vi "Main IU.vi"() -> ()   [LabVIEW 2019]
panel:
  out "Numeric":dbl
  in  "RESET 2":bool
  in  "Tiempo 2":dbl
  in  "Tiempo 1":dbl
  in  "Home":bool
  in  "Aceleración final Motor 2":dbl
  in  "Aceleración final Motor 1":dbl
  in  "Velocidad final Motor 2":dbl
  in  "Velocidad final Motor 1":dbl
  out "String":string
  in  "GO 2":bool
  in  "Aceleración inicial Motor 2":dbl
  in  "Aceleración inicial Motor 1":dbl
  in  "Velocidad inicial Motor 2":dbl
  in  "Velocidad inicial Motor 1":dbl
  in  "RESET 1":bool
  in  "Trayectoria":bool
  in  "GO":bool
  in  "Posición final Motor 2":dbl
  in  "MOTORES INDEPENDIENTES":bool
  in  "Tab Control":enum32{"Motor 1", "Motor 2"}(tab)
  out "Waveform Chart 6":waveform(dbl)[](graph)
  out "Waveform Chart 5":waveform(dbl)[](graph)
  out "Hall 1":bool
  out "Hall 2":bool
  out "Waveform Chart 4":waveform(dbl)[](graph)
  out "Waveform Chart 3":waveform(dbl)[](graph)
  out "Hall 2":bool
  out "Waveform Chart 2":waveform(dbl)[](graph)
  out "Hall1":bool
  in  "Stop UI and RT":bool
  in  "Stop UI":bool
  in  "Posición final motor 1":dbl
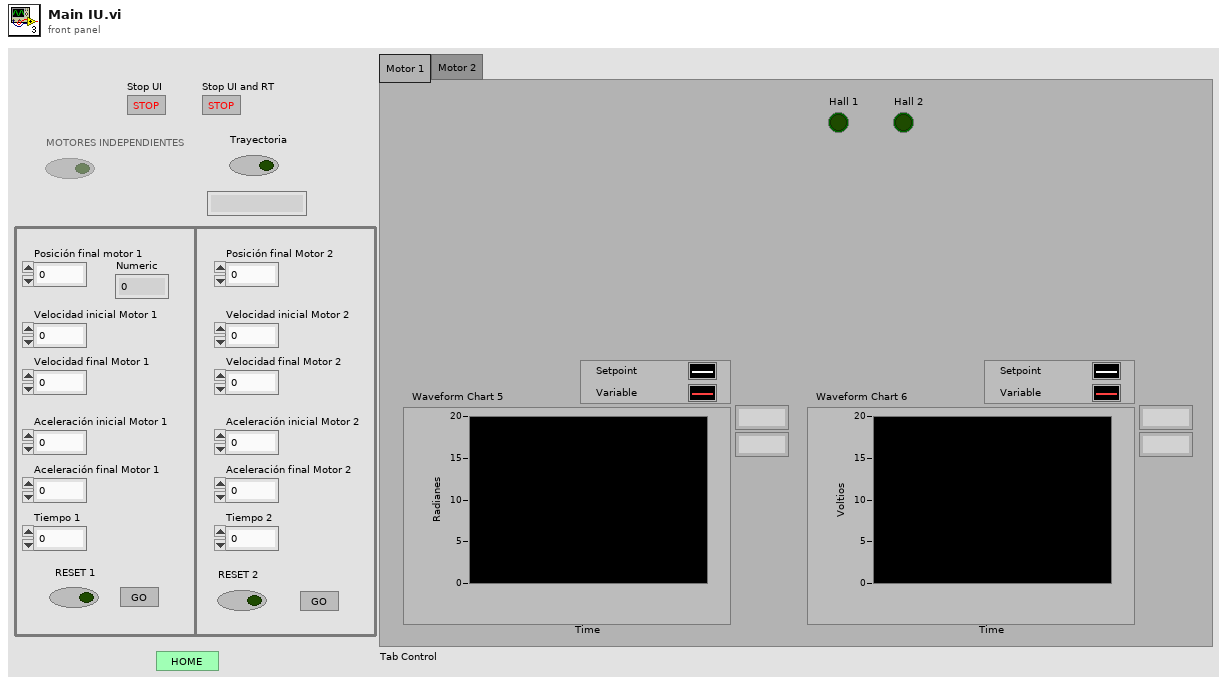
[diagram p1: front panel]
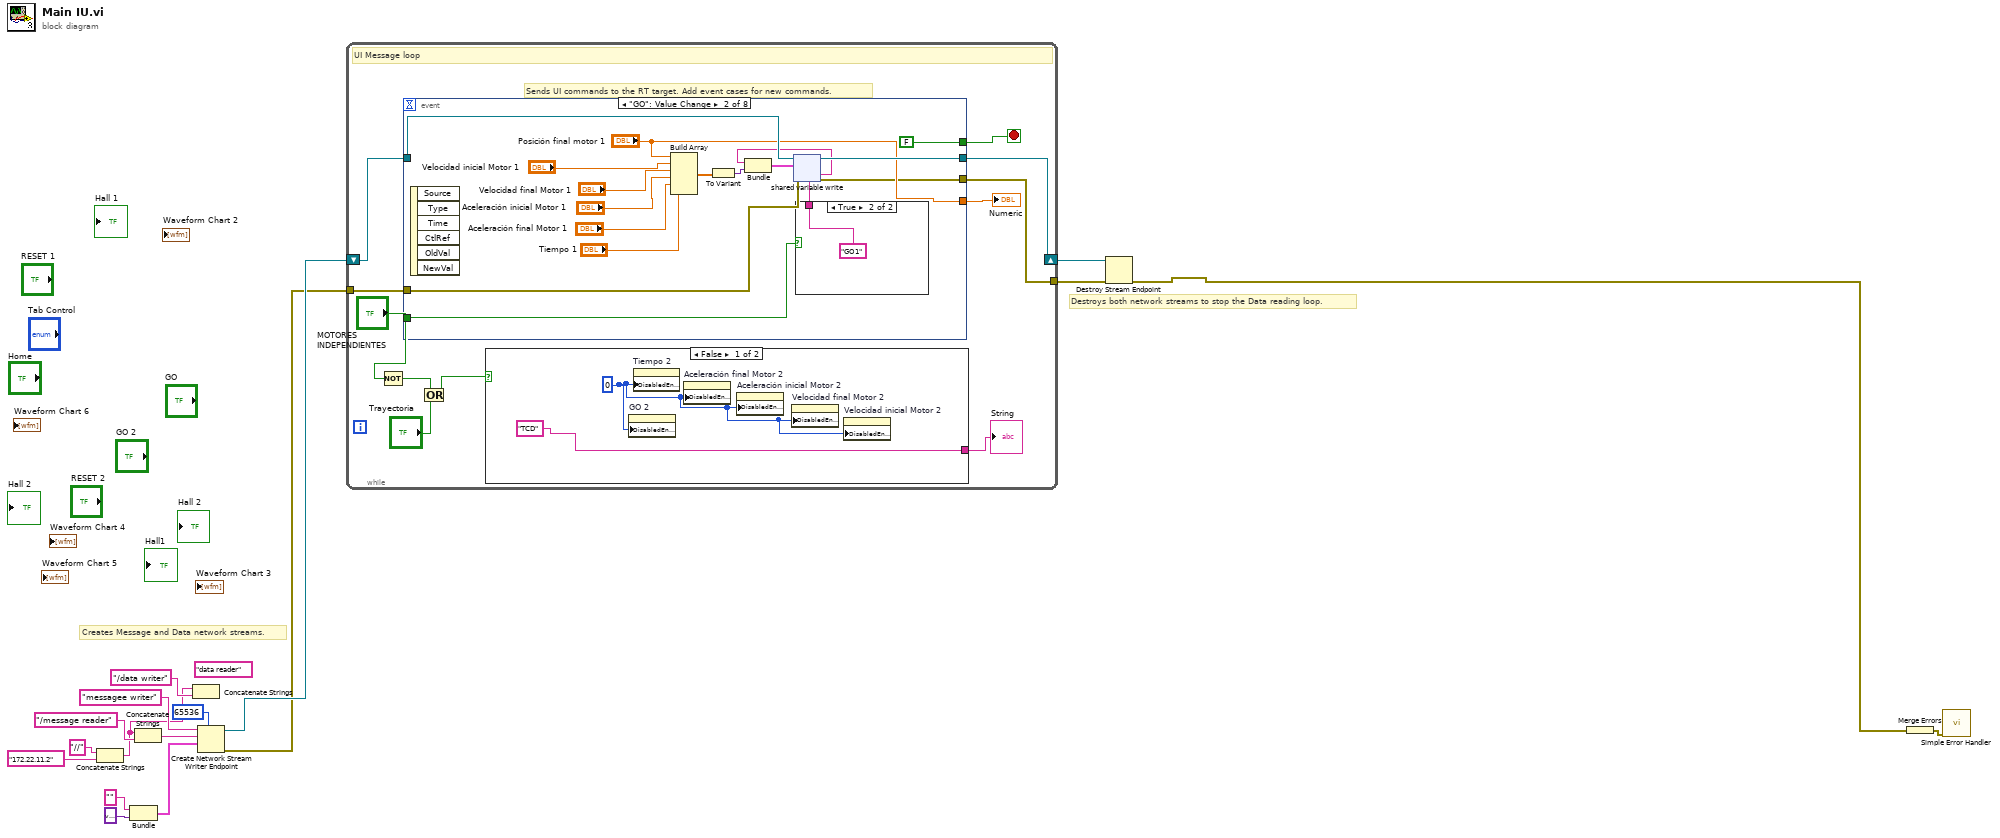
[diagram p0: block diagram]
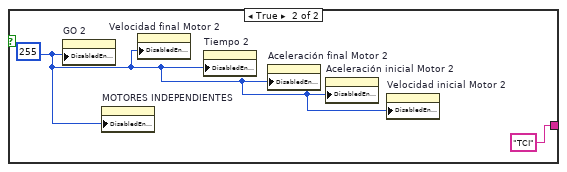
[diagram p2: hidden frame]
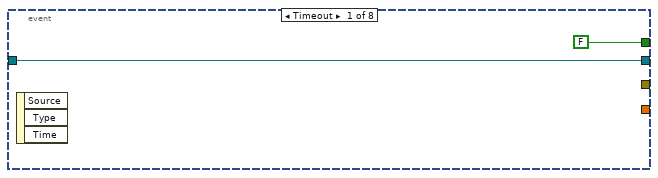
[diagram p3: hidden frame]
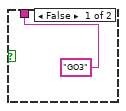
[diagram p4: hidden frame]
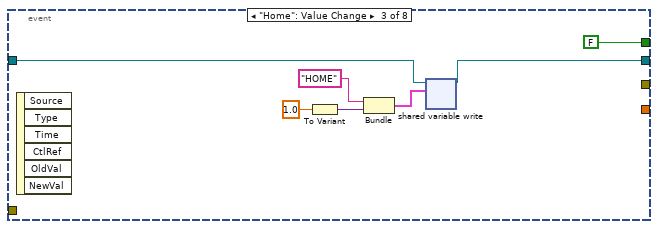
[diagram p5: hidden frame]
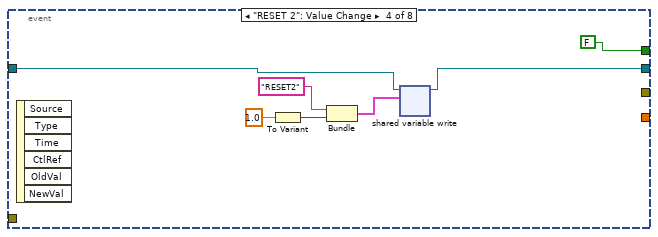
[diagram p6: hidden frame]
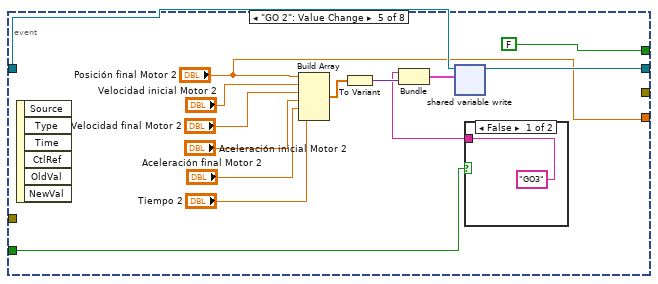
[diagram p7: hidden frame]
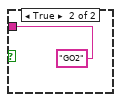
[diagram p8: hidden frame]
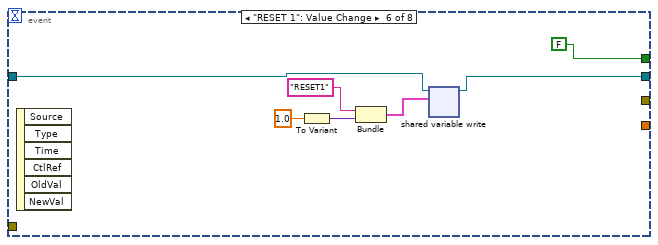
[diagram p9: hidden frame]
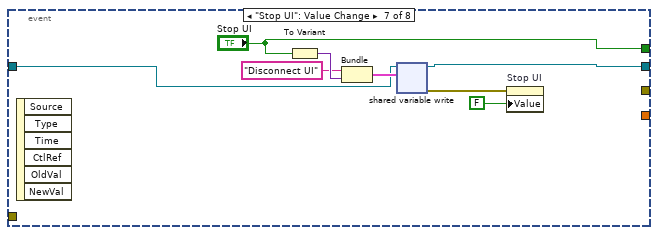
[diagram p10: hidden frame]
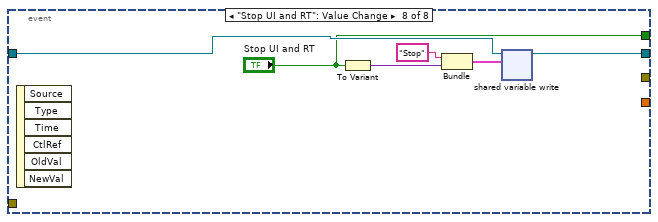
[diagram p11: hidden frame]
diagram:
  (unwired) "data reader" ("reader name")
  # "Destroys both network streams to stop the Data reading loop."
  # "Creates Message and Data network streams."
  n1 = Concatenate Strings("//", "172.22.11.2" ("myRIO IP")) -> (w4:string)
  n2 = Bundle("", variant) -> (w17:cluster{string, variant})  [unwired: 1 in]
  n3 = Concatenate Strings(w4, "/message reader") -> (w5:string)
  n4 = Concatenate Strings(w4, "/data writer") -> ()  [unwired: 1 out]
  n5 = Create Network Stream Writer Endpoint(7:65536 ("writer buffer size"), 9:w17, 10:w5, 11:"messagee writer" ("writer name")) -> (0:w1:errorcluster, 3:w11:refnum<k21>)  [unwired: 3 in]
  n6 = while {
    shift-right: [w27] -> w7
    shift-left: w11 -> [w28]
    tunnel: [w19] -> w2
    tunnel: w1 -> [w18]
    stop <- w26 stop-if-true
    # "Sends UI commands to the RT target. Add event cases for new commands."
    # "UI Message loop"
    n7 = Not(x="MOTORES INDEPENDIENTES") -> (.not. x?=w24:bool)
    n8 = event shown="[1] \"GO\": Value Change" {
      selector: _ -> [_ _ _ _ _ _ _ _]
      dyn-events: _ -> [_ _ _ _ _ _ _ _]
      timeout: _ -> [_ _ _ _ _ _ _ _]
      tunnel: w28 -> [w34 w50 w56 w61 w77 w84 w94 w99]
      tunnel: [w34 w47 w55 w62 w78 w85 w93 w100] -> w27
      tunnel: [FALSE ("Stop UI and RT") FALSE ("Stop UI and RT") FALSE FALSE ("Stop UI and RT") FALSE ("Stop UI and RT") FALSE ("Stop UI and RT") "Stop UI" "Stop UI and RT"] -> w26
      tunnel: "MOTORES INDEPENDIENTES" -> [_ w42 _ _ w69 _ _ _]
      tunnel: [_ "Posición final motor 1" _ _ "Posición final Motor 2" _ _ _] -> w20
      tunnel: [_ w36 _ _ _ _ _ _] -> w19
      tunnel: w18 -> [_ w35 _ _ _ _ _ _]
      event Timeout {
        n9 = event-data() -> ()  [unwired: 1 in, 3 out]
      }
      event "GO": Value Change {
        n10 = event-data() -> ()  [unwired: 1 in, 6 out]
        n11 = Build Array("Posición final motor 1", "Velocidad inicial Motor 1", "Velocidad final Motor 1", "Aceleración inicial Motor 1", "Aceleración final Motor 1", "Tiempo 1") -> (w44:dbl[])
        n12 = To Variant(anything=w44) -> (Variant=w49:variant)
        n13 = case shown="True" w42 {
          tunnel: ["GO3" ("writer name") "GO1" ("writer name")] -> w45
          frame False {
          }
          frame True {
          }
        }
        n14 = Bundle("writer name"=w45, "Variant"=w49) -> (w48:cluster{"writer name":string, "Variant":variant})  [unwired: 1 in]
        n15 = shared-variable-write(w50, w35, w48) -> (w47:refnum<k21>, w36:errorcluster)  [unwired: 1 in, 1 out]
      }
      event "Home": Value Change {
        n16 = event-data() -> ()  [unwired: 1 in, 6 out]
        n17 = To Variant(anything=1.0) -> (Variant=w59:variant)
        n18 = Bundle("writer name"="HOME", "Variant"=w59) -> (w57:cluster{"writer name":string, "Variant":variant})  [unwired: 1 in]
        n19 = shared-variable-write(w56, w57) -> (w55:refnum<k21>)  [unwired: 2 in, 2 out]
      }
      event "RESET 2": Value Change {
        n20 = event-data() -> ()  [unwired: 1 in, 6 out]
        n21 = To Variant(anything=1.0) -> (Variant=w65:variant)
        n22 = Bundle("writer name"="RESET2", "Variant"=w65) -> (w66:cluster{"writer name":string, "Variant":variant})  [unwired: 1 in]
        n23 = shared-variable-write(w61, w66) -> (w62:refnum<k21>)  [unwired: 2 in, 2 out]
      }
      event "GO 2": Value Change {
        n24 = event-data() -> ()  [unwired: 1 in, 6 out]
        n25 = Build Array("Posición final Motor 2", "Velocidad inicial Motor 2", "Velocidad final Motor 2", "Aceleración inicial Motor 2", "Aceleración final Motor 2", "Tiempo 2") -> (w75:dbl[])
        n26 = To Variant(anything=w75) -> (Variant=w80:variant)
        n27 = case shown="False" w69 {
          tunnel: ["GO3" ("writer name") "GO2" ("writer name")] -> w68
          frame False {
          }
          frame True {
          }
        }
        n28 = Bundle("writer name"=w68, "Variant"=w80) -> (w79:cluster{"writer name":string, "Variant":variant})  [unwired: 1 in]
        n29 = shared-variable-write(w77, w79) -> (w78:refnum<k21>)  [unwired: 2 in, 2 out]
      }
      event "RESET 1": Value Change {
        n30 = event-data() -> ()  [unwired: 1 in, 6 out]
        n31 = To Variant(anything=1.0) -> (Variant=w88:variant)
        n32 = Bundle("writer name"="RESET1", "Variant"=w88) -> (w89:cluster{"writer name":string, "Variant":variant})  [unwired: 1 in]
        n33 = shared-variable-write(w84, w89) -> (w85:refnum<k21>)  [unwired: 2 in, 2 out]
      }
      event "Stop UI": Value Change {
        n34 = event-data() -> ()  [unwired: 1 in, 6 out]
        n35 = To Variant(anything="Stop UI") -> (Variant=w97:variant)
        n36 = Bundle("writer name"="Disconnect UI", "Variant"=w97) -> (w96:cluster{"writer name":string, "Variant":variant})  [unwired: 1 in]
        n37 = shared-variable-write(w94, w96) -> (w93:refnum<k21>, w90:errorcluster)  [unwired: 2 in, 1 out]
        n38 = property on="Stop UI" class="Bool (strict)"(error in=w90, "Value"=FALSE ("Stop UI and RT")) -> ()  [unwired: 1 in, 2 out]
      }
      event "Stop UI and RT": Value Change {
        n39 = event-data() -> ()  [unwired: 1 in, 6 out]
        n40 = To Variant(anything="Stop UI and RT") -> (Variant=w103:variant)
        n41 = Bundle("writer name"="Stop", "Variant"=w103) -> (w102:cluster{"writer name":string, "Variant":variant})  [unwired: 1 in]
        n42 = shared-variable-write(w99, w102) -> (w100:refnum<k21>)  [unwired: 2 in, 2 out]
      }
    }
    "Numeric" <- w20
    n43 = Or(x=w24, y="Trayectoria") -> (x .or. y?=w23:bool)
    n44 = case shown="False" w23 {
      tunnel: ["TCD" "TCI"] -> w21
      frame False {
        w29 = 0
        n45 = property on="GO 2" class="Bool"("DisabledEnum"=w29) -> ()  [unwired: 2 in, 2 out]
        n46 = property on="Tiempo 2" class="DigNum (strict)"("DisabledEnum"=w29) -> ()  [unwired: 2 in, 2 out]
        n47 = property on="Aceleración final Motor 2" class="DigNum (strict)"("DisabledEnum"=w29) -> ()  [unwired: 2 in, 2 out]
        n48 = property on="Aceleración inicial Motor 2" class="DigNum (strict)"("DisabledEnum"=w29) -> ()  [unwired: 2 in, 2 out]
        n49 = property on="Velocidad final Motor 2" class="DigNum (strict)"("DisabledEnum"=w29) -> ()  [unwired: 2 in, 2 out]
        n50 = property on="Velocidad inicial Motor 2" class="DigNum (strict)"("DisabledEnum"=w29) -> ()  [unwired: 2 in, 2 out]
      }
      frame True {
        w31 = 255
        n51 = property on="GO 2" class="Bool"("DisabledEnum"=w31) -> ()  [unwired: 2 in, 2 out]
        n52 = property on="MOTORES INDEPENDIENTES" class="Bool (strict)"("DisabledEnum"=w31) -> ()  [unwired: 2 in, 2 out]
        n53 = property on="Velocidad final Motor 2" class="DigNum (strict)"("DisabledEnum"=w31) -> ()  [unwired: 2 in, 2 out]
        n54 = property on="Tiempo 2" class="DigNum (strict)"("DisabledEnum"=w31) -> ()  [unwired: 2 in, 2 out]
        n55 = property on="Aceleración final Motor 2" class="DigNum (strict)"("DisabledEnum"=w31) -> ()  [unwired: 2 in, 2 out]
        n56 = property on="Aceleración inicial Motor 2" class="DigNum (strict)"("DisabledEnum"=w31) -> ()  [unwired: 2 in, 2 out]
        n57 = property on="Velocidad inicial Motor 2" class="DigNum (strict)"("DisabledEnum"=w31) -> ()  [unwired: 2 in, 2 out]
      }
    }
    "String" <- w21
  }
  n58 = Destroy Stream Endpoint(8:w2, 11:w7) -> (0:w3:errorcluster)
  n59 = Merge Errors(w3) -> (w8:errorcluster)
  n60 = call <vilib>:"Simple Error Handler.vi"("error in (no error)"=w8) -> ()  [unwired: 4 in, 5 out]
